vi "Sample_Finite_InfiniteTrigger.vi"() -> ()   [LabVIEW 2013]
doc: "This samples demonstrates how to sample a finite waveform."
uses:
  <userlib>/ArtScope/Trigger/ArtScope_ConfigureTriggerEdge.vi
  <userlib>/ArtScope/Fetch/ArtScope_FetchBinary16.vi
  <userlib>/ArtScope/_SubVI/ArtScope_ArrayByChannel_U16.vi
panel:
  out "error out":errorcluster
  in  "reference position":dbl
  in  "sensitive":i32=50
  in  "coupling":i32(ring) items=["DC", "AC", "HIG", "LOW"]
  in  "count":i32
  in  "slope":i32(ring) items=["下降", "上升", "变化"]
  in  "source":string(combo)="VAL_TRIGGER_CH0"
  in  "level(mV)":dbl=1000.0
  in  "range(Vpp)":i32(ring)=1 items=["20V", "10V", "2V", "40V", "16V", "8V", "4V", "1.6V", "800m", "400m", "160m", "80m", "40m"]
  in  "offset(mV)":i32
  in  "NumSamples":i32=10240
  in  "Stop":bool
  out "waveform":u16[][](graph)
  in  "Timeout(s)":dbl=10.0
  in  "MinRecordLength":i32=10240
  in  "MinSampleRate":dbl=4000000.0
  in  "Coupling":i32(ring) items=["DC", "AC"]
  in  "Channel Name":string="0"
  in  "Resource Name":string="Dev5"
  # "Vertical"
  # "Horizontal"
  # "Trigger"
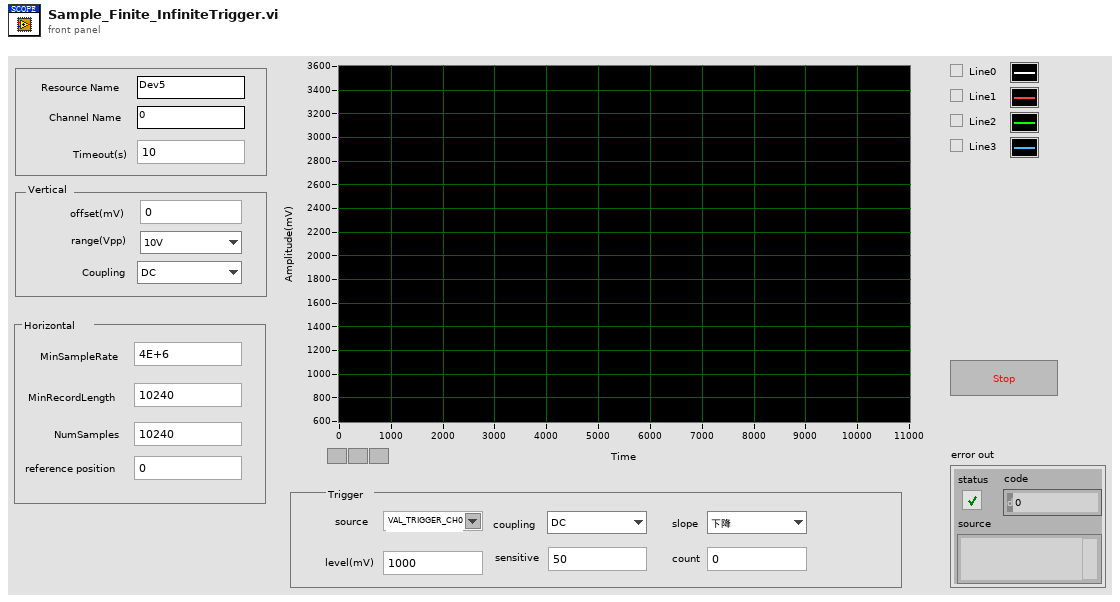
[diagram p1: front panel]
types:
  T1 = cluster{"fLSB":cluster{dbl, dbl, dbl, dbl, dbl, dbl, dbl, dbl}, "RangeValue":cluster{dbl, dbl, dbl, dbl, dbl, dbl, dbl, dbl}, "wMaxLSB":u32, "TriggerMode":i32, "sampLengthPerChan":u32, "pAvailSampsPoints":u32, "channelCount":i32}
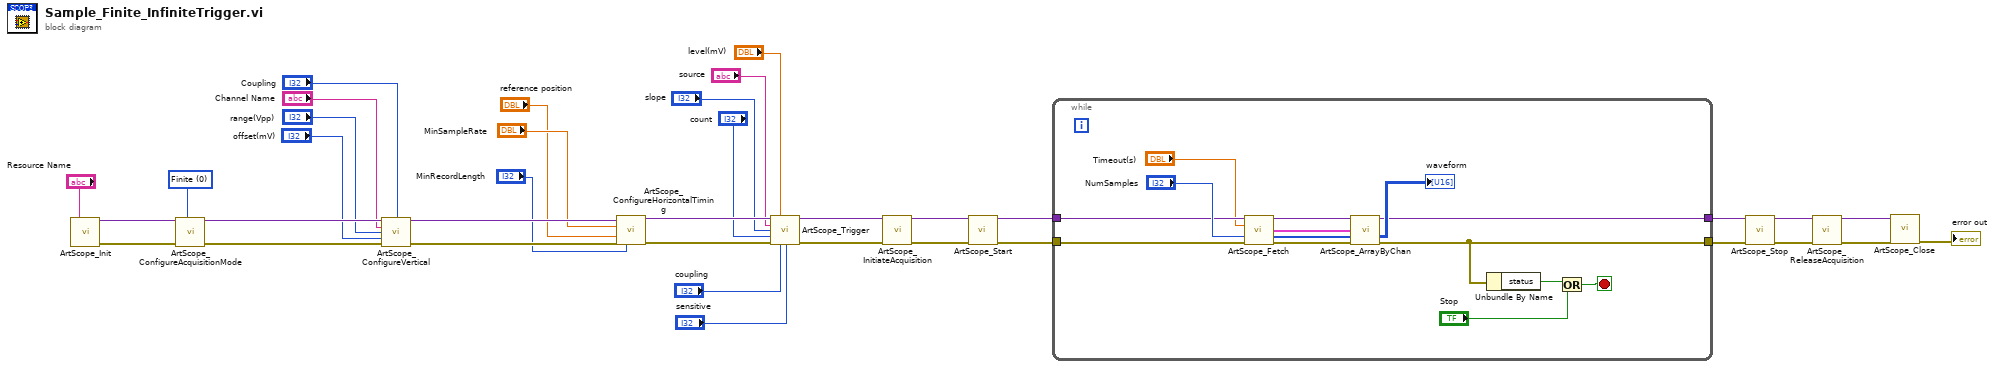
[diagram p0: block diagram]
diagram:
  w29 = 0 items=["Finite", "Continuous"] ("AcuqMode")
  n1 = call <userlib>:"ArtScope_Init.vi"("task name"="Resource Name") -> ("task handle"=w30:variant, "error out"=w31:errorcluster)  [unwired: 13 in]
  n2 = call <userlib>:"ArtScope_ConfigureAcquisitionMode.vi"("task handle"=w30, "acquisition mode"=w29, "error in (no error)"=w31) -> ("task handle"=w28:variant, "error out"=w32:errorcluster)  [unwired: 11 in]
  n3 = call <userlib>:"ArtScope_ConfigureVertical.vi"("task handle"=w28, "coupling"="Coupling", "channels"="Channel Name", "range(Vpp)"="range(Vpp)", "offset"="offset(mV)", "error in (no error)"=w32) -> ("task handle"=w34:variant, "error out"=w33:errorcluster)  [unwired: 8 in]
  n4 = call <userlib>:"ArtScope_ConfigureHorizontalTiming.vi"("task handle"=w34, "min sample rate"="MinSampleRate", "reference position"="reference position", "error in (no error)"=w33, "min record length"="MinRecordLength") -> ("task handle"=w26:variant, "error out"=w27:errorcluster)  [unwired: 9 in]
  n5 = call-poly <userlib>:"ArtScope_Trigger.vi"("task handle"=w26, "level"="level(mV)", "trigger source"="source", "slope"="slope", "trigger count"="count", "error in (no error)"=w27, "trigger coupling"="coupling", "trigger sensitive"="sensitive") -> ("task handle"=w20:variant, "error out"=w19:errorcluster)  [unwired: 6 in]
  n6 = call <userlib>:"ArtScope_InitiateAcquisition.vi"("task handle"=w20, "error in (no error)"=w19) -> ("task handle"=w9:variant, "error out"=w8:errorcluster)  [unwired: 12 in]
  n7 = call <userlib>:"ArtScope_Start.vi"("task handle"=w9, "error in (no error)"=w8) -> ("task handle"=w7:variant, "error out"=w6:errorcluster)  [unwired: 12 in]
  n8 = while {
    tunnel: w7 -> [w41]
    tunnel: w6 -> [w42]
    tunnel: [w39] -> w5
    tunnel: [w38] -> w3
    stop <- w50 stop-if-true
    n9 = call-poly <userlib>:"ArtScope_Fetch.vi"("task handle"=w41, "timeout"="Timeout(s)", "num samples"="NumSamples", "error in (no error)"=w42) -> ("task handle"=w46:variant, "wfm info"=w45:T1, "data"=w44:u16[], "error out"=w47:errorcluster)  [unwired: 8 in]
    n10 = call-poly <userlib>:"ArtScope_ArrayByChan.vi"("task handle"=w46, "wfm info"=w45, "1D data"=w44, "error in (no error)"=w47) -> ("task handle"=w39:variant, "2D data"=→"waveform":u16[][], "error out"=w38:errorcluster)  [unwired: 9 in]
    n11 = Unbundle By Name(w38) -> ("status"=w37:bool)
    n12 = Or(x=w37, y="Stop") -> (x .or. y?=w50:bool)
  }
  n13 = call <userlib>:"ArtScope_Stop.vi"("task handle"=w5, "error in (no error)"=w3) -> ("task handle"=w4:variant, "error out"=w2:errorcluster)  [unwired: 12 in]
  n14 = call <userlib>:"ArtScope_ReleaseAcquisition.vi"("task handle"=w4, "error in (no error)"=w2) -> ("task handle"=w22:variant, "error out"=w21:errorcluster)  [unwired: 12 in]
  n15 = call <userlib>:"ArtScope_Close.vi"("task handle"=w22, "error in (no error)"=w21) -> ("error out"=→"error out":errorcluster)  [unwired: 13 in]
